vi "sound.vi"() -> ()   [LabVIEW 2012]
panel:
  out "Waveform Chart":dbl(graph)
  out "Numeric":dbl
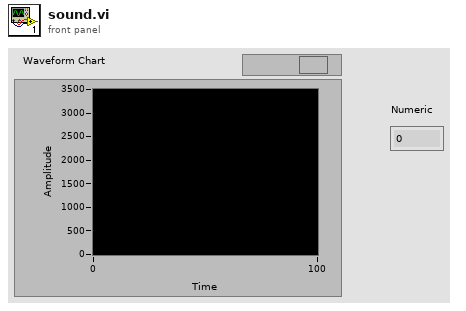
[diagram p1: front panel]
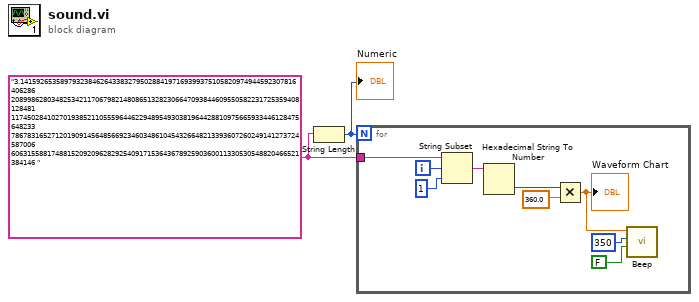
[diagram p0: block diagram]
diagram:
  w1 = "3.141592653589793238462643383279502884197169399375105820974944592307816406286 208998628034825342117067982148086513282306647093844609550582231725359408128481 117450284102701938521105559644622948954930381964428810975665933446128475648233 786783165271201909145648566923460348610454326648213393607260249141273724587006 606315588174881520920962829254091715364367892590360011330530548820466521384146 "
  n1 = String Length(string=w1) -> (length=w2:i32)
  "Numeric" <- w2
  n2 = for {
    N: w2 -> [_]
    tunnel: w1 -> [w8]
    i -> [w7]
    n3 = String Subset(string=w8, offset (0)=w7, length (rest)=1 ("length (rest)")) -> (substring=w4:string)
    n4 = Hexadecimal String To Number(string=w4) -> (number=w3:u32)  [unwired: 2 in, 1 out]
    n5 = Multiply(x=w3, y=360.0) -> (x*y=w5:dbl)
    "Waveform Chart" <- w5
    n6 = call <vilib>:"Beep.vi"("use system alert? (T)"=FALSE, "duration (msec)"=u32 350, "frequency (Hz)"=w5) -> ()  [unwired: 9 in]
  }
